vi "Handle Last Ack Core.vi"(4 "error in (no error)":errorcluster, 6 "Last Ack":refnum<class "Last Ack.lvclass">, 7 "PersistantConnectionHandler in":refnum<class "PersistantConnectionHandler.lvclass">) -> (0 "error out":errorcluster, 3 "PersistantConnectionHandler out":refnum<class "PersistantConnectionHandler.lvclass">)   [LabVIEW 2020, in "PersitantConnectionHandler.lvlib" / "PersistantConnectionHandler.lvclass"]
doc: "(<B>Filename</B>: Actor Framework.lvlib:Actor.lvclass:Handle Last Ack Core.vi)\n\nDefines how the caller actor responds to the Last Ack message from a nested actor. The Last Ack message is the final message a nested actor sends to its caller before it shuts down. The message contains information about the final state of the nested actor.\n\nBy default, this method does nothing except return any error the nested actor sent. A descendant class may override this method to define behavior."
uses:
  <vilib>/gpm_packages/@cs/Network-interface/Source/PersistantConnectionHandler/PersistantConnectionHandler/PersistantConnectionHandler.lvclass
  <vilib>/ActorFramework/LastAck/Last Ack.lvclass
  C:/Program Files/National Instruments/LabVIEW 2020/vi.lib/gpm_packages/@cs/Network-interface/Source/Logged Actor/LoggedActor.lvclass
  <vilib>/gpm_packages/@cs/Network-interface/Source/Connection Reference/Connection Reference/Connection Reference.lvclass
  <vilib>/gpm_packages/@cs/event-logger/Source/Composed Log/Types/Log Level.ctl
  <vilib>/ActorFramework/LastAck/Last Ack.lvclass/Last Ack.ctl
  <vilib>/gpm_packages/@cs/Network-interface/Source/PersistantConnectionHandler/PersistantConnectionHandler/PersistantConnectionHandler.lvclass/PersistantConnectionHandler.ctl
  <vilib>/gpm_packages/@cs/Network-interface/Source/Logged Actor/LoggedActor.lvclass/LoggedActor.ctl
  <vilib>/gpm_packages/@cs/event-logger/Source/Composed Log/LoggerReference/LoggerReference.lvclass/LoggerReference.ctl
  <vilib>/gpm_packages/@cs/event-logger/Source/Composed Log/LoggerReference/Log Event.vi
  <vilib>/gpm_packages/@cs/event-logger/Source/Composed Log/LoggerReference/Log.vi
  <vilib>/gpm_packages/@cs/event-logger/Source/Composed Log/LoggerReference/Get Valid Event Time.vi
  <vilib>/gpm_packages/@cs/event-logger/Source/Composed Log/LoggerReference/Remove Stale Logs.vi
  <vilib>/gpm_packages/@cs/Network-interface/Source/MessagingInterfaces/IConnectionStateChangeCallback/IConnectionStateChangeCallback.lvclass
  <vilib>/gpm_packages/@cs/Network-interface/Source/Logged Actor/LoggedActor.lvclass
  <vilib>/gpm_packages/@cs/event-logger/Source/Composed Log/Composed Log.lvlib
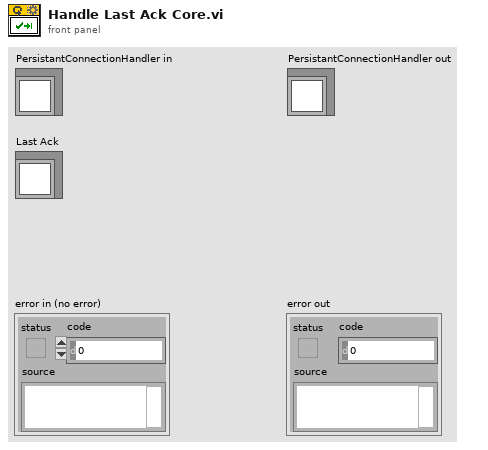
[diagram p1: front panel]
types:
  T1 = typedef "Composed Log.lvlib/Log Level.ctl" = enum16{"Debug", "Info", "Warning", "Error", "Critical"}
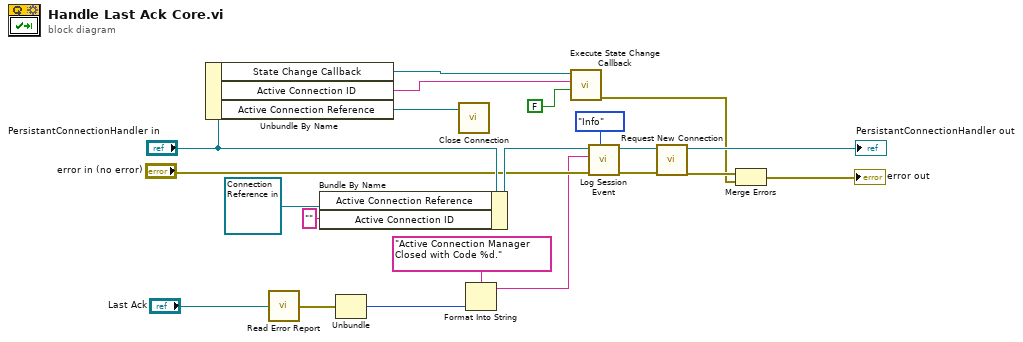
[diagram p0: block diagram]
diagram:
  n1 = Unbundle By Name("PersistantConnectionHandler in") -> ("State Change Callback"=w16:refnum<class "IConnectionStateChangeCallback.lvclass">, "Active Connection ID"=w15:string, "Active Connection Reference"=w21:refnum<data-value>)
  n2 = call <vilib>:"Read Error Report.vi"("Last Ack"="Last Ack") -> ("error report"=w5:errorcluster)
  n3 = Bundle By Name(cluster="PersistantConnectionHandler in", "Active Connection Reference"=refnum<data-value> refnum, "Active Connection ID"="") -> (w10:refnum<class "PersistantConnectionHandler.lvclass">)
  n4 = Unbundle(w5) -> ("code"=w4:i32)  [unwired: 2 out]
  n5 = call <vilib>:"Close Connection.vi"("Connection Reference In"=w21) -> ()  [unwired: 10 in, 1 out]
  n6 = Format Into String(format string="Active Connection Manager Closed with Code %d.", w4) -> (resulting string=w2:string)  [unwired: 2 in, 1 out]
  n7 = call-dynamic "Execute State Change Callback.vi"("Connection State"=FALSE, "Connection ID"=w15, "IConnectionStateChangeCallback in"=w16) -> ("error out"=w12:errorcluster)  [unwired: 8 in]
  n8 = call <vilib>:"Log Session Event.vi"("Event Level"=Log_Level."Info", "error in (no error)"="error in (no error)", "Event Data"=w2, "SessionActor in"=w10) -> ("error out"=w7:errorcluster, "SessionActor out"=w8:refnum<class "PersistantConnectionHandler.lvclass">)  [unwired: 6 in]
  n9 = call <vilib>:"Request New Connection.vi"("error in (no error)"=w7, "PersistantConnectionHandler in"=w8) -> ("error out"=w18:errorcluster, "PersistantConnectionHandler out"=→"PersistantConnectionHandler out":refnum<class "PersistantConnectionHandler.lvclass">)  [unwired: 8 in]
  n10 = Merge Errors(w18, w12) -> (→"error out":errorcluster)
